vi "Transform_Create_TransRot.vi"(9 "ROTATION":T3, 11 "TRANSLATION":T2) -> (3 "TRANSFORM":T1)   [LabVIEW 2019, in "PathExecution_Library.lvlib"]
uses:
  TRANSLATION.ctl
  ROTATION.ctl
  TRANSFORM.ctl
  PathExecution_Library.lvlib
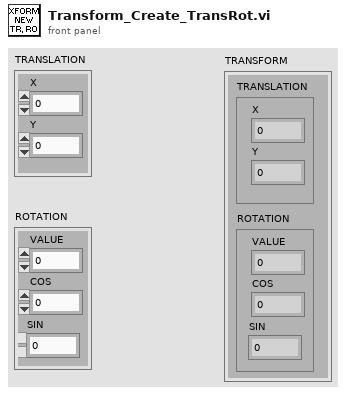
[diagram p1: front panel]
types:
  T1 = typedef "PathExecution_Library.lvlib/TRANSFORM.ctl" = cluster{"TRANSLATION":T2, "ROTATION":T3}
  T2 = typedef "PathExecution_Library.lvlib/TRANSLATION.ctl" = cluster{"X":dbl, "Y":dbl}
  T3 = typedef "PathExecution_Library.lvlib/ROTATION.ctl" = cluster{"VALUE":dbl, "COS":dbl, "SIN":dbl}
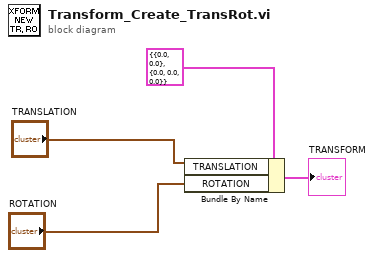
[diagram p0: block diagram]
diagram:
  n1 = Bundle By Name(cluster=T1 {"TRANSLATION"={"X"=0.0, "Y"=0.0}, "ROTATION"={"VALUE"=0.0, "COS"=0.0, "SIN"=0.0}} ("TRANSFORM"), "TRANSLATION"="TRANSLATION", "ROTATION"="ROTATION") -> (→"TRANSFORM":T1)
